vi "Drive Get.vi"(1 "Joystick In":T1) -> (0 "Get Out":T2)   [LabVIEW 2016]
uses:
  <vilib>/Rock Robotics/WPI/Ultrasonic/WPI_SonarSRF04DigitalRefNum Registry Get.vi
  <vilib>/Rock Robotics/WPI/Ultrasonic/WPI_SonarSRF04DigitalGetRange.vi
  <vilib>/Rock Robotics/Network Tables/NT Write Number.vi
panel:
  in  "Sensitivity":dbl
  in  "Reset":bool
  in  "acc":dbl
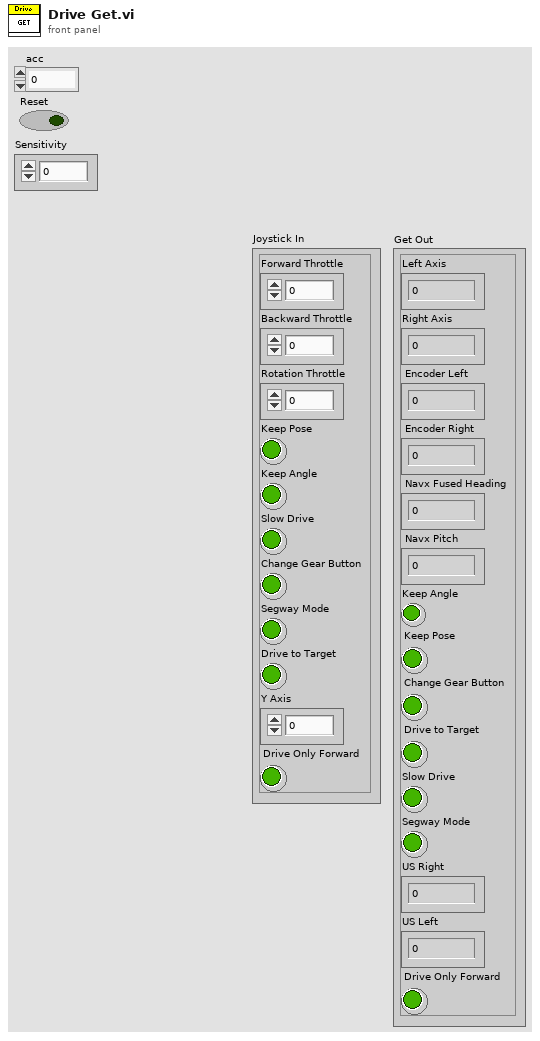
[diagram p1: front panel]
types:
  T1 = cluster{"Forward Throttle":dbl, "Backward Throttle":dbl, "Rotation Throttle":dbl, "Keep Pose":bool, "Keep Angle":bool, "Slow Drive":bool, "Change Gear Button":bool, "Segway Mode":bool, "Drive to Target":bool, "Y Axis":dbl, "Drive Only Forward":bool}
  T2 = cluster{"Left Axis":dbl, "Right Axis":dbl, " Encoder Left":dbl, " Encoder Right":dbl, " Navx Fused Heading":dbl, " Navx Pitch":dbl, "Keep Angle":bool, "Keep Pose":bool, "Change Gear Button":bool, "Drive to Target":bool, "Slow Drive":bool, "Segway Mode":bool, "US Right":dbl, "US Left":dbl, "Drive Only Forward":bool}
  T3 = cluster{"Yaw":dbl, "Roll":dbl, "Pitch":dbl, "Heading":dbl, "Fused Heading":dbl}
  T4 = typedef "WPI_UltrasonicDeviceRef.ctl" = cluster{"DevStatus":errorcluster, "Ping Channel":T5, "Echo Channel":T5, "CntIndex":T6}
  T5 = typedef "FPGA_DIOChannel.ctl" = enum8{"DIO 0", "DIO 1", "DIO 2", "DIO 3", "DIO 4", "DIO 5", "DIO 6", "DIO 7", "DIO 8", "DIO 9", "DIO MXP 0", "DIO MXP 1", "DIO MXP 2", "DIO MXP 3", "DIO MXP 4", "DIO MXP 5", "DIO MXP 6", "DIO MXP 7", "DIO MXP 8", "DIO MXP 9", "DIO MXP 10", "DIO MXP 11", "DIO MXP 12", "DIO MXP 13", "DIO MXP 14", "DIO MXP 15", "SPI Port CS1", "SPI Port CS2", "SPI Port CS3", "SPI Port MISO", "SPI Port MOSI", "Invalid"}
  T6 = typedef "FPGA_CounterCtrSystemIndex.ctl" = enum8{"Ctr 0", "Ctr 1", "Ctr 2", "Ctr 3", "Ctr 4", "Ctr 5", "Ctr 6", "Ctr 7", "Invalid"}
  T7 = typedef "WPI_EncoderDevRef.ctl" = cluster{"DevStatus":errorcluster, "EncoderIndex":T8, "CounterIndex":T6, "DistancePerCount":dbl, "Decoding Type":T9}
  T8 = typedef "FPGA_EncoderIdx.ctl" = enum8{"Enc 0", "Enc 1", "Enc 2", "Enc 3", "Enc 4", "Enc 5", "Enc 6", "Enc 7", "Invalid"}
  T9 = typedef "WPI_EncoderType.ctl" = enum16{"1x", "2x", "4x"}
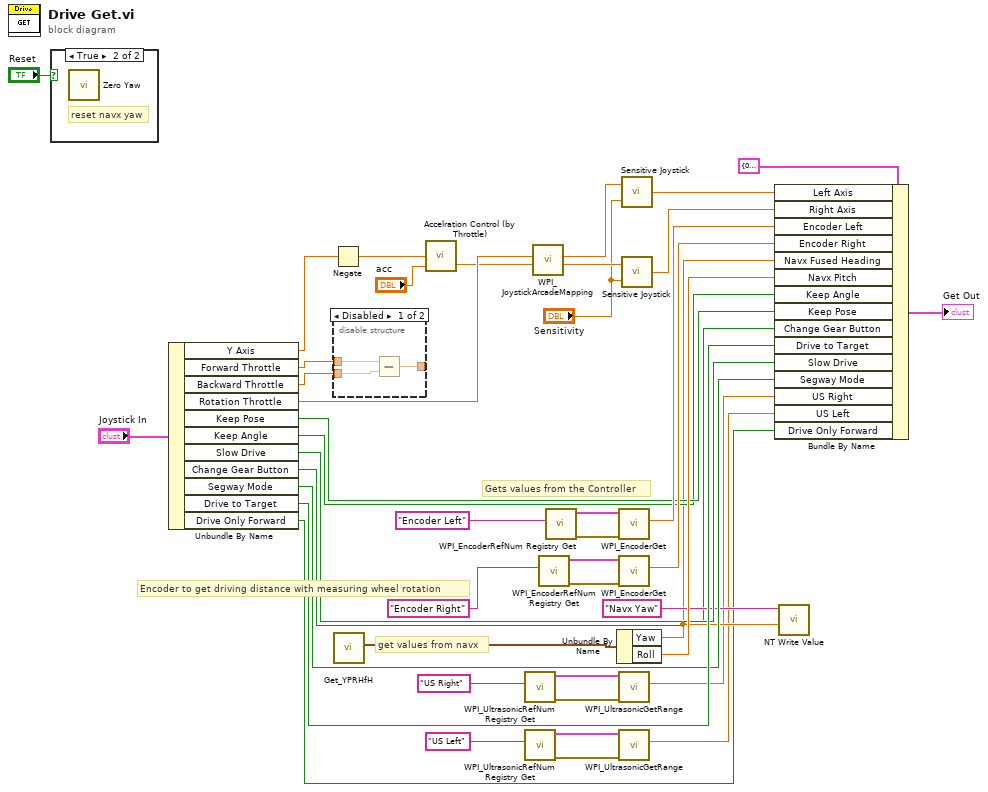
[diagram p0: block diagram]
diagram:
  # "get values from navx"
  # "Encoder to get driving distance with measuring wheel rotation"
  # "Gets values from the Controller"
  n1 = case shown="True" "Reset" {
    frame False {
    }
    frame True {
      # "reset navx yaw"
      n2 = call <vilib>:"Zero Yaw.vi"() -> ()  [unwired: 12 in]
    }
  }
  n3 = Unbundle By Name("Joystick In") -> ("Y Axis"=w22:dbl, "Forward Throttle"=w35:dbl, "Backward Throttle"=w34:dbl, "Rotation Throttle"=w25:dbl, "Keep Pose"=w30:bool, "Keep Angle"=w29:bool, "Slow Drive"=w27:bool, "Change Gear Button"=w12:bool, "Segway Mode"=w26:bool, "Drive to Target"=w28:bool, "Drive Only Forward"=w1:bool)
  n4 = Negate(x=w22) -> (-x=w16:dbl)
  n5 = disable-structure shown="Disabled" {
    disable-tunnel: w35 -> [w46 _]
    disable-tunnel: w34 -> [w45 _]
    disable-tunnel: [w44 _] -> _
    frame Disabled {
      n6 = Subtract(x=w46, y=w45) -> (x-y=w44:dbl)
    }
    frame Enabled {
    }
  }
  n7 = call <vilib>:"Get_YPRHfH.vi"() -> ("YRPHfH"=w13:T3)  [unwired: 11 in]
  n8 = call "Accelration Control (by Throttle).vi"("acc"="acc", "Yinput"=w16) -> ("Youtput"=w23:dbl)  [unwired: 1 in, 1 out]
  n9 = call-poly <vilib>:"WPI_UltrasonicRefNum Registry Get.vi"("refnum name"="US Right") -> ("error out"=w9:errorcluster, "SonarSRF04DevRef"=w8:T4)  [unwired: 9 in]
  n10 = call-poly <vilib>:"WPI_UltrasonicRefNum Registry Get.vi"("refnum name"="US Left") -> ("error out"=w11:errorcluster, "SonarSRF04DevRef"=w10:T4)  [unwired: 9 in]
  n11 = call <vilib>:"WPI_JoystickArcadeMapping.vi"("Y axis value"=w23, "X axis value"=w25) -> ("Right Motor Value"=w19:dbl, "Left Motor Value"=w21:dbl)  [unwired: 8 in]
  n12 = call <vilib>:"WPI_EncoderRefNum Registry Get.vi"("refnum name"="Encoder Right") -> ("error out"=w42:errorcluster, "EncoderDevRef"=w43:T7)  [unwired: 9 in]
  n13 = call <vilib>:"WPI_EncoderRefNum Registry Get.vi"("refnum name"="Encoder Left") -> ("error out"=w40:errorcluster, "EncoderDevRef"=w38:T7)  [unwired: 9 in]
  n14 = Unbundle By Name(w13) -> ("Yaw"=w14:dbl, "Roll"=w31:dbl)
  n15 = call <vilib>:"WPI_EncoderGet.vi"("error in (no error)"=w40, "EncoderDevRef"=w38) -> ("Distance"=w33:dbl)  [unwired: 4 in, 5 out]
  n16 = call <vilib>:"WPI_EncoderGet.vi"("error in (no error)"=w42, "EncoderDevRef"=w43) -> ("Distance"=w32:dbl)  [unwired: 4 in, 5 out]
  n17 = call-poly <vilib>:"WPI_UltrasonicGetRange.vi"("error in (no error)"=w9, "SonarSRF04DevRef"=w8) -> ("Distance"=w5:dbl)  [unwired: 7 in, 2 out]
  n18 = call-poly <vilib>:"WPI_UltrasonicGetRange.vi"("error in (no error)"=w11, "SonarSRF04DevRef"=w10) -> ("Distance"=w4:dbl)  [unwired: 7 in, 2 out]
  n19 = call "Sensitive Joystick.vi"("Sensitivity"="Sensitivity", "Joystick In"=w21) -> ("Joystick Out"=w20:dbl)
  n20 = call "Sensitive Joystick.vi"("Sensitivity"="Sensitivity", "Joystick In"=w19) -> ("Joystick Out"=w17:dbl)
  n21 = Bundle By Name(cluster=T2 {"Left Axis"=0.0, "Right Axis"=0.0, " Encoder Left"=0.0, " Encoder Right"=0.0, " Navx Fused Heading"=0.0, " Navx Pitch"=0.0, "Keep Angle"=FALSE, "Keep Pose"=FALSE, "Change Gear Button"=FALSE, "Drive to Target"=FALSE, "Slow Drive"=FALSE, "Segway Mode"=FALSE, "US Right"=0.0, "US Left"=0.0, "Drive Only Forward"=FALSE} ("Get Out"), "Left Axis"=w20, "Right Axis"=w17, "Encoder Left"=w33, "Encoder Right"=w32, "Navx Fused Heading"=w14, "Navx Pitch"=w31, "Keep Angle"=w29, "Keep Pose"=w30, "Change Gear Button"=w12, "Drive to Target"=w28, "Slow Drive"=w27, "Segway Mode"=w26, "US Right"=w5, "US Left"=w4, "Drive Only Forward"=w1) -> (→"Get Out":T2)
  n22 = call-poly <vilib>:"NT Write Value.vi"("Numeric"=w14, "Name"="Navx Yaw") -> ()  [unwired: 9 in, 1 out]
